vi "PolarToRect.vi"(6 "Scan Info":T1 {"delay" format="%.3f"; "pivot distance" format="%.2f"; "sector scan angle" format="%.2f"}, 9 "Time between pt\nmicros":dbl format="%.2f", 10 "c m/s":dbl=1500.0, 11 "array dims":i32[](array[numeric])) -> (1 "y":dbl[][](array[numeric]) format="%.2f", 2 "x":dbl[][](array[numeric]) format="%.2f", 3 "# lines per scan":u16, 4 "sector scan angle":sgl format="%.2f", 5 "# rf points per line":u16, 7 "polar axis":cluster{"r axis":dbl[], "theta axis":dbl[]} {"theta axis" format="%.2f"; "r axis" format="%.2f"})   [LabVIEW 2022 SP3]
uses:
  <vilib>/Analysis/NI_AALPro.lvlib
panel:
  out "r":dbl[][](array[numeric]) format="%.4f"
  out "theta":dbl[][](array[numeric]) format="%.5e"
  # "Can feed x y and z into a\n3-D surface plot to get a nice sector \nimage view."
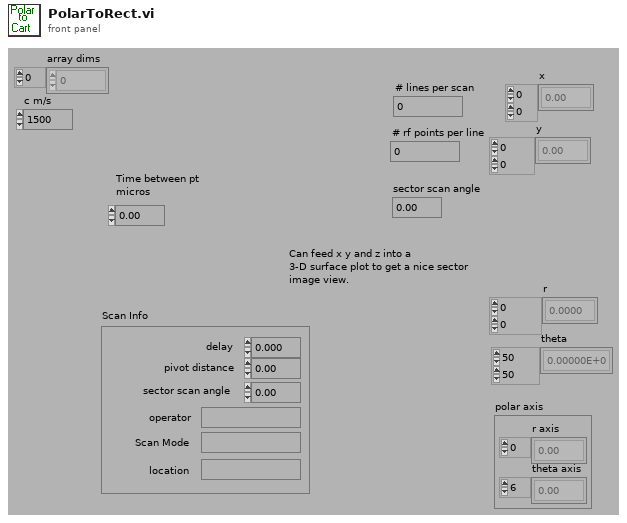
[diagram p1: front panel]
types:
  T1 = cluster{"delay":sgl, "pivot distance":sgl, "sector scan angle":sgl, "operator":string, "Scan Mode":string, "location":string}
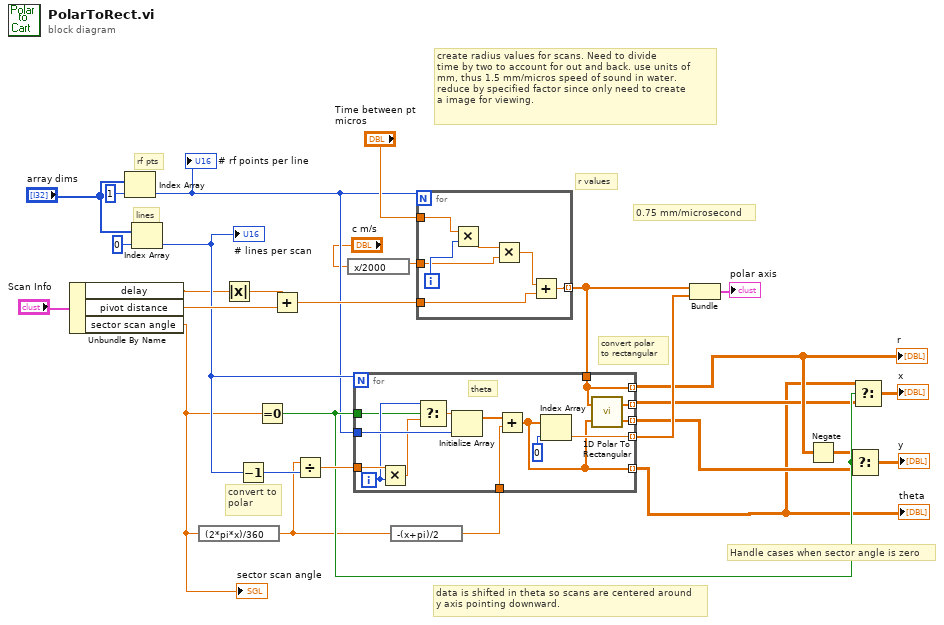
[diagram p0: block diagram]
diagram:
  # "convert polar\nto rectangular"
  # "Handle cases when sector angle is zero"
  # "0.75 mm/microsecond"
  # "lines"
  # "rf pts"
  # "create radius values for scans. Need to divide \ntime by two to account for out and back. use units of\nmm, thus 1.5 mm/micros speed of sound in water.\nreduce by specified factor since only need to create\na image for viewing."
  # "r values"
  # "convert to\npolar"
  # "data is shifted in theta so scans are centered around\ny axis pointing downward."
  n1 = Unbundle By Name("Scan Info") -> ("delay"=w5:sgl, "pivot distance"=w24:sgl, "sector scan angle"=w11:sgl)
  "sector scan angle" <- w11
  n2 = Index Array(array="array dims", index=1 ("Index")) -> (element=w3:i32)
  "# rf points per line" <- w3
  n3 = Index Array(array="array dims", index=0 ("Index")) -> (element=w23:i32)
  "# lines per scan" <- w23
  n4 = expression code="(2*pi*x)/360"(w11) -> (w10:sgl)
  n5 = Absolute Value(x=w5) -> (abs(x)=w13:sgl)
  n6 = Decrement(x=w23) -> (x-1=w19:i32)
  n7 = Equal To 0?(x=w11) -> (x = 0?=w15:bool)
  n8 = Add(x=w13, y=w24) -> (x+y=w29:sgl)
  n9 = Divide(x=w10, y=w19) -> (x/y=w28:sgl)
  n10 = expression code="x/2000"("c m/s") -> (w1:dbl)
  n11 = expression code="-(x+pi)/2"(w10) -> (w12:sgl)
  n12 = for {
    N: w3 -> [_]
    tunnel: w29 -> [w36]
    tunnel: [w35] -> w18 mode=indexing
    tunnel: "Time between pt\nmicros" -> [w34]
    tunnel: w1 -> [w30]
    i -> [w31]
    n13 = Multiply(x=w34, y=w31) -> (x*y=w33:dbl)
    n14 = Multiply(x=w33, y=w30) -> (x*y=w32:dbl)
    n15 = Add(x=w32, y=w36) -> (x+y=w35:dbl)
  }
  n16 = for {
    N: w23 -> [_]
    tunnel: w28 -> [w50]
    tunnel: w18 -> [w40]
    tunnel: w3 -> [w49]
    tunnel: w12 -> [w48]
    tunnel: [w46] -> w21 mode=indexing
    tunnel: [w39] -> w6 mode=indexing
    tunnel: [w40] -> w9 mode=indexing
    tunnel: w15 -> [w41]
    tunnel: [w38] -> w8 mode=indexing
    tunnel: [w37] -> w7 mode=indexing
    i -> [w44]
    # "theta"
    n17 = Multiply(x=w50, y=w44) -> (x*y=w45:sgl)
    n18 = Select(t=w44, s=w41, f=w45) -> (s? t:f=w43:sgl)
    n19 = Initialize Array(w43, w49) -> (w42:sgl[])
    n20 = Add(x=w42, y=w48) -> (x+y=w39:sgl[])
    n21 = Index Array(array=w39, index=0) -> (element=w46:sgl)
    n22 = call <vilib>:"1D Polar To Rectangular.vi"("Magnitude"=w40, "Phase"=w39) -> ("X"=w38:dbl[], "Y"=w37:dbl[])  [unwired: 1 out]
  }
  "theta" <- w6
  "r" <- w9
  n23 = Bundle(w18, w21) -> (→"polar axis":cluster{dbl[], sgl[]})  [unwired: 1 out]
  n24 = Negate(x=w9) -> (-x=w14:dbl[][])
  n25 = Select(t=w14, s=w15, f=w7) -> (s? t:f=→"y":dbl[][])
  n26 = Select(t=w6, s=w15, f=w8) -> (s? t:f=→"x":dbl[][])
